vi "Target Dimensions info + Seen now.vi"(0 "Target 1 Height":dbl, 1 "Target 1 Width":dbl, 2 "Target 1 Height from ground to center":dbl, 3 "Target 2 Height":dbl, 4 "Target 2 Width":dbl, 5 "Target 2 Height from ground to center":dbl, 6 "Real life height":dbl, 7 "Target 3 Height":dbl, 9 "Target 3 Width":dbl, 11 "Target 3 Height from ground to center":dbl) -> (15 "Target num":i32, 16 "Target Height from ground to center":dbl, 17 "Target Height":dbl, 18 "Target Width":dbl)   [LabVIEW 2012]
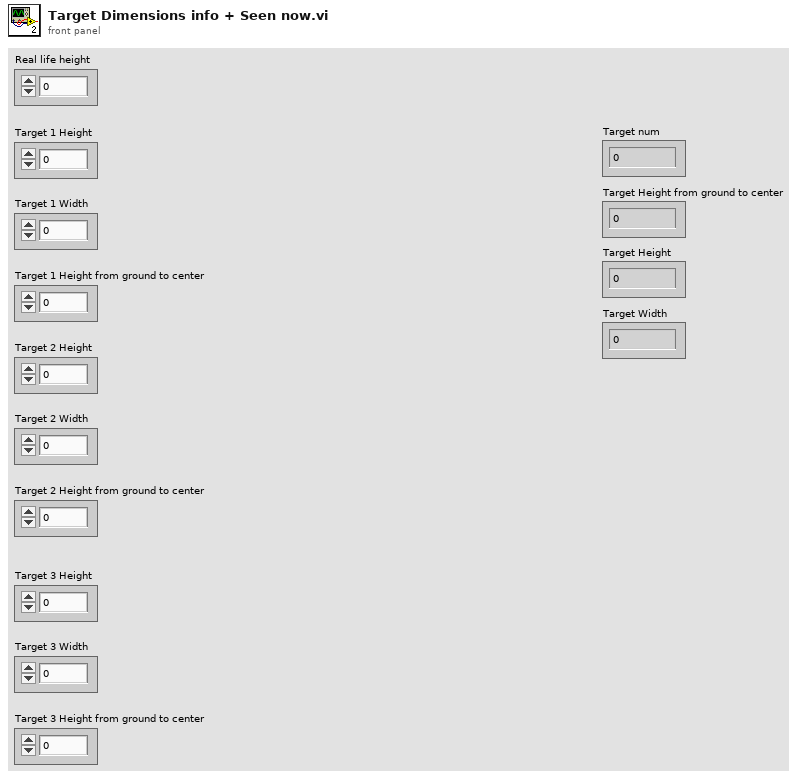
[diagram p1: front panel]
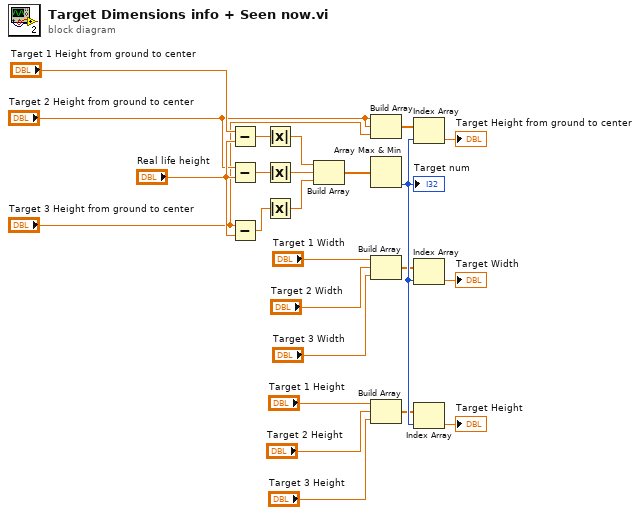
[diagram p0: block diagram]
diagram:
  n1 = Subtract(x="Target 1 Height from ground to center", y="Real life height") -> (x-y=w20:dbl)
  n2 = Subtract(x="Target 2 Height from ground to center", y="Real life height") -> (x-y=w19:dbl)
  n3 = Subtract(x="Target 3 Height from ground to center", y="Real life height") -> (x-y=w18:dbl)
  n4 = Absolute Value(x=w20) -> (abs(x)=w17:dbl)
  n5 = Absolute Value(x=w19) -> (abs(x)=w16:dbl)
  n6 = Absolute Value(x=w18) -> (abs(x)=w15:dbl)
  n7 = Build Array(w17, w16, w15) -> (w24:dbl[])
  n8 = Build Array("Target 2 Height from ground to center", "Target 2 Height from ground to center", "Target 3 Height from ground to center") -> (w8:dbl[])
  n9 = Array Max & Min(array=w24) -> (min index (indices)=w23:i32)  [unwired: 3 out]
  "Target num" <- w23
  n10 = Build Array("Target 1 Width", "Target 2 Width", "Target 3 Width") -> (w7:dbl[])
  n11 = Build Array("Target 1 Height", "Target 2 Height", "Target 3 Height") -> (w9:dbl[])
  n12 = Index Array(array=w8, index=w23) -> (element=→"Target Height from ground to center":dbl)
  n13 = Index Array(array=w7, index=w23) -> (element=→"Target Width":dbl)
  n14 = Index Array(array=w9, index=w23) -> (element=→"Target Height":dbl)
